vi "SF2_BUFFER.vi"(9 "Buffer Time (sec)":dbl=10.0 format="%#_13g", 11 "Sample rate":u8=50) -> ()   [LabVIEW 2016]
uses:
  _Process_Loop/FRIC_SF2_Process Loop TypeDef.ctl
  _Process_Loop/FRIC_SF2_ProcessingLoopStatesTypeDef_I2C.ctl
  _Notifier/SF2_NotifyPacketTypeDef.ctl
  _Notifier/SF2_ActionTypeDef.ctl
  <vilib>/Platform/TimedLoop/XDataNode/timing_clust.ctl
  <vilib>/Platform/TimedLoop/XDataNode/nitl_modes.ctl
  <vilib>/Platform/TimedLoop/XDataNode/wakeup.ctl
  <vilib>/Platform/TimedLoop/XDataNode/XDataNode.xnode
  <vilib>/Platform/TimedLoop/XDataNode/XDNodeRunTimeDep.lvlib
panel:
  out "Buffer Full":bool
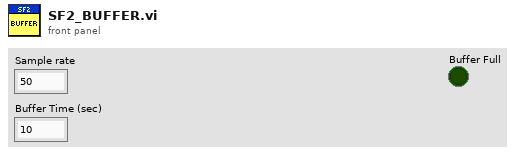
[diagram p1: front panel]
types:
  T1 = typedef "FRIC_SF2_Process Loop TypeDef.ctl" = cluster{"State Array":T2[], "error":errorcluster, "SF2 Buffer":dbl[][], "Loop Frequency":u32, "Buffer Size":dbl, "notifier ref out":refnum<notifier>, "Sample rate":u8}
  T2 = typedef "FRIC_SF2_ProcessingLoopStatesTypeDef_I2C.ctl" = enum16{"Process", "Hault", "Exit", "VI_INI"}
  T3 = typedef "XDNodeRunTimeDep.lvlib/timing_clust.ctl" = cluster{"Expected End [f-1]":u64, "Actual End [f-1]":u64, "Finished Late? [f-1]":bool, "Expected End [i-1]":u64, "Actual End [i-1]":u64, "Finished Late? [i-1]":bool, "Expected Start [i]":u64, "Actual Start [i]":u64, "Expected Start [f]":u64, "Actual Start [f]":u64, "Source Name":string, "Structure Name":string, "Period":i64, "Deadline":i64, "Offset":i64, "Start":i64, "Priority":i32, "Timeout":i32, "Mode":T4, "Wakeup Reason":T5, "Error":errorcluster, "Source Type":string, "Secondary Source Type":string, "Global End Time":u64, "Global Start Time":u64, "Frame Duration":u64, "Iteration Duration":u64, "Assigned CPU":i32, "I/O Scan Engine Mode":u32}
  T4 = typedef "XDNodeRunTimeDep.lvlib/nitl_modes.ctl" = enum32{"No Change", "Process missed periods, maintain original phase", "Discard missed periods, maintain original phase", "Process missed periods, ignore original phase", "Discard missed periods, ignore original phase"}
  T5 = typedef "XDNodeRunTimeDep.lvlib/wakeup.ctl" = enum32{"Normal", "Aborted", "Asynchronous wakeup", "Timing source error", "Timed loop error", "Timeout"}
  T6 = typedef "SF2_NotifyPacketTypeDef.ctl" = cluster{"SF2 Action":T7, "Data":variant}
  T7 = typedef "SF2_ActionTypeDef.ctl" = enum16{"None", "Halt", "Reset Buffer"}
  T8 = cluster{"Quat W":dbl, "Quat X":dbl, "Quat Y":dbl, "Quat Z":dbl}
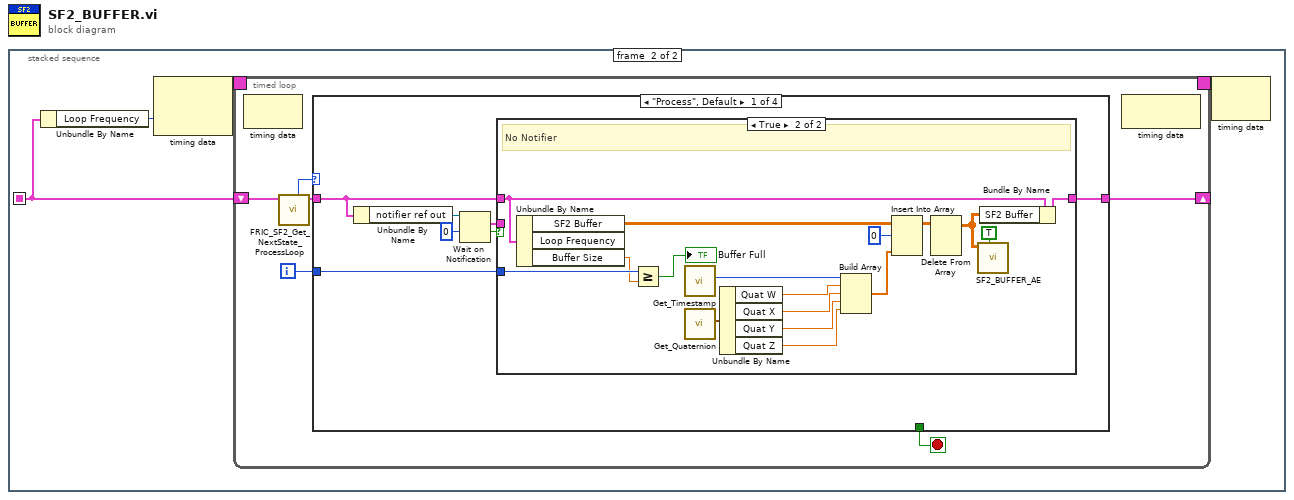
[diagram p0: block diagram]
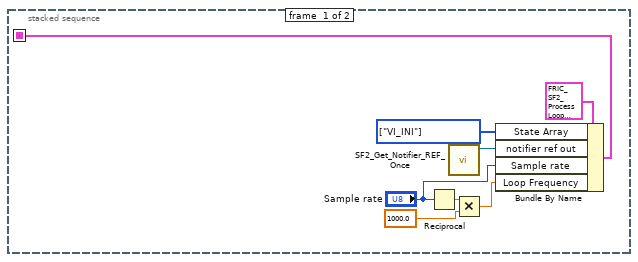
[diagram p2: hidden frame]
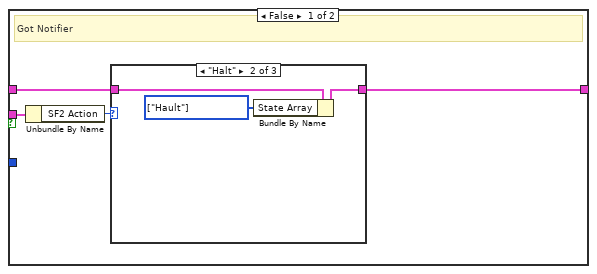
[diagram p3: hidden frame]
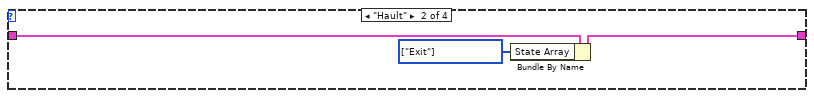
[diagram p6: hidden frame]
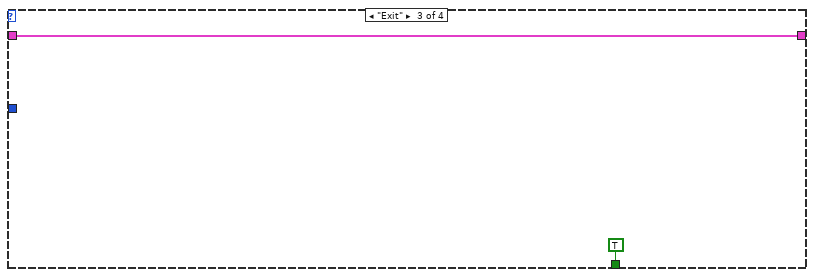
[diagram p7: hidden frame]
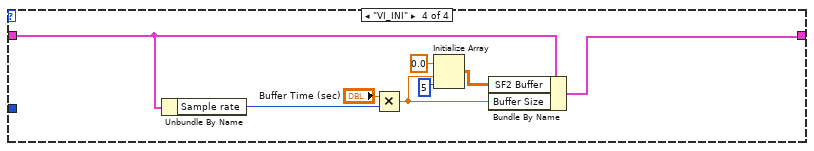
[diagram p8: hidden frame]
diagram:
  n1 = stacked-sequence {
    seq-local: [w7 _] -> [_ w10]
    frame #0 {
      w5 = T2[] [enum."VI_INI"] items=["Process", "Hault", "Exit", "VI_INI"] ("State Array")
      n2 = Reciprocal(x="Sample rate") -> (1/x=w4:dbl)
      n3 = call "SF2_Get_Notifier_REF_Once.vi"() -> ("notifier ref out"=w6:refnum<notifier>)  [unwired: 10 in, 1 out]
      n4 = Multiply(x=w4, y=1000.0) -> (x*y=w2:dbl)
      n5 = Bundle By Name(cluster=T1 {"State Array"=[enum."Hault", enum."Process"], "error"={"status"=FALSE, "code"=0, "source"=""}, "SF2 Buffer"=[], "Loop Frequency"=200, "Buffer Size"=2000.0, "notifier ref out"=refnum, "Sample rate"=200} ("SF2 Process Loop TypeDef (out)"), "State Array"=w5, "notifier ref out"=w6, "Sample rate"="Sample rate", "Loop Frequency"=w2) -> (w7:T1)
    }
    frame #1 {
      n6 = Unbundle By Name(w10) -> ("Loop Frequency"=w9:u32)
      n7 = node-c288(w9) -> (w12:T3)  [unwired: 1 in]
      n8 = timed-loop {
        shift-right: [w15] -> _
        shift-left: w10 -> [w17]
        timing: w12 -> [_]
        timing-out: [_] -> w11
        i -> [w14]
        stop <- w18 stop-if-true
        n9 = node-c288() -> ()  [unwired: 1 in, 1 out]
        n10 = call "FRIC_SF2_Get_NextState_ProcessLoop.vi"("SF2 Process Loop TypeDef (in)"=w17) -> ("SF2 Process Loop TypeDef (out)"=w16:T1, "Current State"=w13:T2)  [unwired: 9 in]
        n11 = case shown="\"Process\", Default" w13 {
          tunnel: [_ _ TRUE _] -> w18
          tunnel: w16 -> [w27 w56 w58 w60]
          tunnel: [w26 w55 w58 w65] -> w15
          tunnel: w14 -> [w25 _ _ _]
          frame "Process", Default {
            n12 = Unbundle By Name(w27) -> ("notifier ref out"=w23:refnum<notifier>)
            n13 = Wait on Notification(notifier=w23, timeout in ms (-1)=0) -> (notification=w21:T6, timed out?=w22:bool)  [unwired: 2 in, 2 out]
            n14 = case shown="True" w22 {
              tunnel: [w29 w49] -> w26
              tunnel: w25 -> [_ w39]
              tunnel: w27 -> [w30 w48]
              tunnel: w21 -> [w31 _]
              frame False {
                # "Got Notifier"
                n15 = Unbundle By Name(w31) -> ("SF2 Action"=w28:T7)
                n16 = case shown="\"Halt\"" w28 {
                  tunnel: w30 -> [w32 w35 w36]
                  tunnel: [w32 w34 w36] -> w29
                  frame "None", Default {
                  }
                  frame "Halt" {
                    w33 = T2[] [enum."Hault"] items=["Process", "Hault", "Exit", "VI_INI"] ("State Array")
                    # "Got Notifier"
                    n17 = Bundle By Name(cluster=w35, "State Array"=w33) -> (w34:T1)
                  }
                  frame "Reset Buffer" {
                  }
                }
              }
              frame True {
                # "No Notifier"
                n18 = Unbundle By Name(w48) -> ("SF2 Buffer"=w50:dbl[][], "Buffer Size"=w38:dbl)  [unwired: 1 out]
                n19 = Greater Or Equal?(x=w39, y=w38) -> (x >= y?=→"Buffer Full":bool)
                n20 = call "Get_Timestamp.vi"() -> ("Timestamp"=w47:u32)  [unwired: 11 in]
                n21 = call "Get_Quaternion.vi"() -> ("Quaternion"=w51:T8)  [unwired: 11 in]
                n22 = Unbundle By Name(w51) -> ("Quat W"=w46:dbl, "Quat X"=w45:dbl, "Quat Y"=w44:dbl, "Quat Z"=w43:dbl)
                n23 = Build Array(w47, w46, w45, w44, w43) -> (w42:dbl[])
                n24 = Insert Into Array(array=w50, index (row)=0 ("index"), new element=w42) -> (w53:dbl[][])  [unwired: 1 in]
                n25 = Delete From Array(array=w53) -> (array with subset deleted=w41:dbl[][])  [unwired: 3 in, 1 out]
                n26 = call "SF2_BUFFER_AE.vi"("Update"=TRUE, "SF2 Buffer (in)"=w41) -> ()  [unwired: 9 in, 1 out]
                n27 = Bundle By Name(cluster=w48, "SF2 Buffer"=w41) -> (w49:T1)
              }
            }
          }
          frame "Hault" {
            w54 = T2[] [enum."Exit"] items=["Process", "Hault", "Exit", "VI_INI"] ("State Array")
            n28 = Bundle By Name(cluster=w56, "State Array"=w54) -> (w55:T1)
          }
          frame "Exit" {
          }
          frame "VI_INI" {
            n29 = Unbundle By Name(w60) -> ("Sample rate"=w59:u8)
            n30 = Multiply(x="Buffer Time (sec)", y=w59) -> (x*y=w62:dbl)
            n31 = Initialize Array(0.0 ("Numeric"), w62, 5 ("dimension size")) -> (w63:dbl[][])
            n32 = Bundle By Name(cluster=w60, "SF2 Buffer"=w63, "Buffer Size"=w62) -> (w65:T1)
          }
        }
        n33 = node-c288() -> ()  [unwired: 1 in, 1 out]
      }
      n34 = node-c288(w11) -> ()  [unwired: 1 out]
    }
  }
